vi "TestLoadImages.vi"() -> ()   [LabVIEW 2022 SP3]
uses:
  <vilib>/vision/NI_Vision_Development_Module.lvlib
panel:
  out "ImageMain 7":T1(plugin-control)
  in  "path":path
  out "ImageMain 6":T1(plugin-control)
  out "ImageMain 5":T1(plugin-control)
  out "ImageMain 4":T1(plugin-control)
  out "ImageMain 3":T1(plugin-control)
  out "ImageMain 2":T1(plugin-control)
  # "M:\\DigiLens-1276\\Printer Recipe Files\\Recipe_Patterns\\CalibrationPrints\\Strip Weights\\IP\\SW_IP2.bmp"
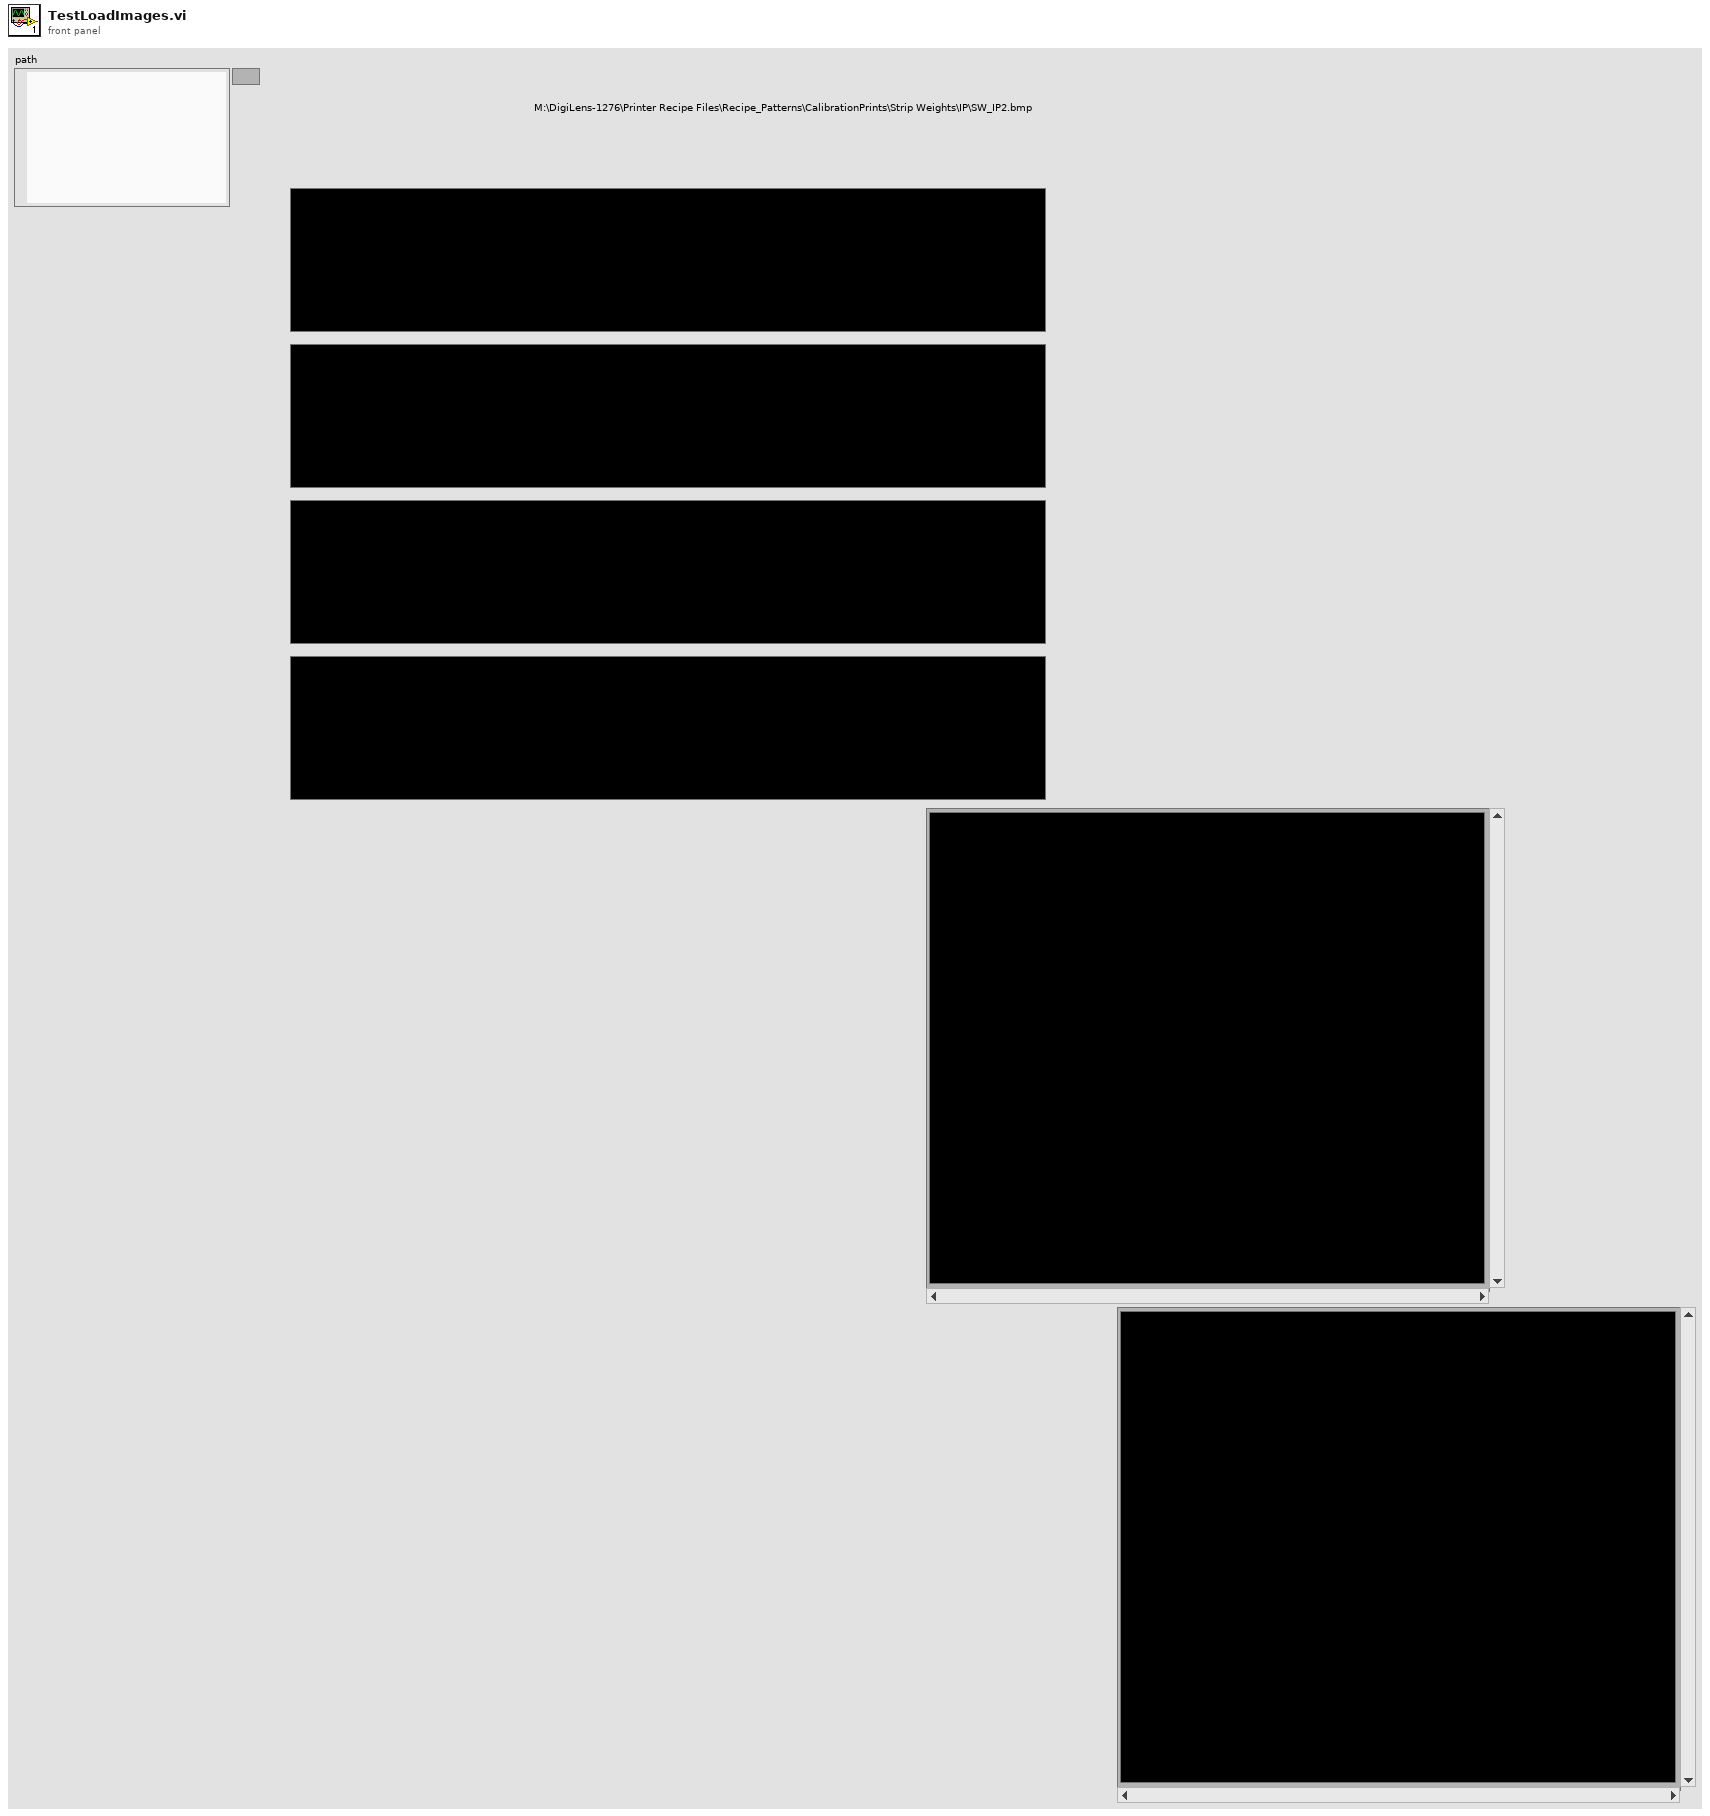
[diagram p1: front panel]
types:
  T1 = typedef "IMAQ Image.ctl" = refnum<image>
  T2 = typedef "Image Type" = u32
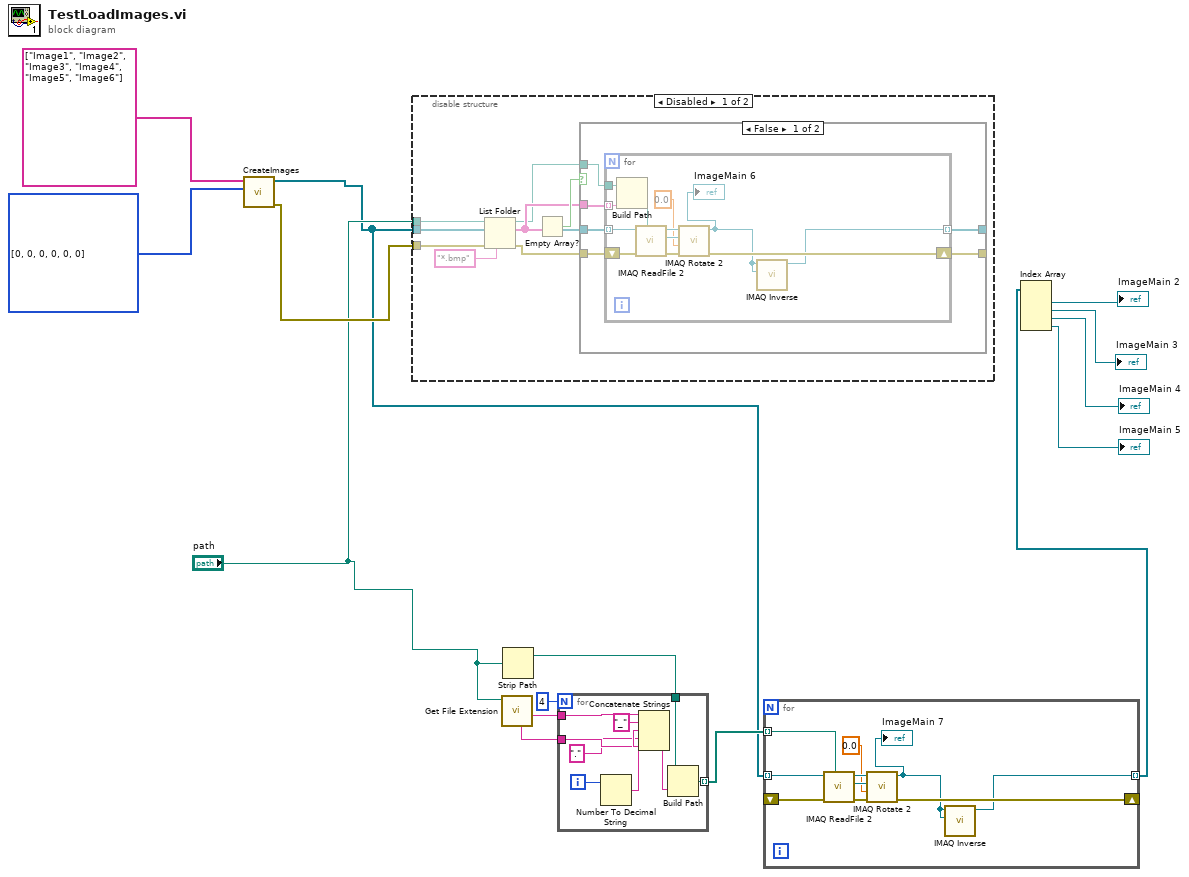
[diagram p0: block diagram]
diagram:
  w15 = T2[] [0, 0, 0, 0, 0, 0] items=["Grayscale (U8)", "Grayscale (I16)", "Grayscale (SGL)", "Complex (CSG)", "RGB (U32)", "HSL (U32)", "RGB (U64)", "Grayscale (U16)"]
  n1 = call "CreateImages.vi"("Array 3"=w15, "Array in"=string[] ["Image1", "Image2", "Image3", "Image4", "Image5", "Image6"]) -> ("error in (no error) 2"=w13:errorcluster, "Array out"=w2:T1[])  [unwired: 8 in]
  n2 = disable-structure shown="Disabled" {
    disable-tunnel: w13 -> [w18 _]
    disable-tunnel: "path" -> [w17 _]
    disable-tunnel: w2 -> [w16 _]
    frame Disabled {
      n3 = List Folder(path=w17, pattern="*.bmp", error in=w18) -> (path out=w19:path, filenames=w21:string[], error out=w20:errorcluster)  [unwired: 1 in, 1 out]
      n4 = Empty Array?(array=w21) -> (empty?=w22:bool)
      n5 = case shown="False" w22 {
        tunnel: w21 -> [w29 _]
        tunnel: w16 -> [w28 w42]
        tunnel: w19 -> [w27 _]
        tunnel: w20 -> [w26 w41]
        tunnel: [w25 w42] -> _
        tunnel: [w24 w41] -> _
        frame False {
          n6 = for {
            tunnel: w29 -> [w40] mode=indexing
            tunnel: w28 -> [w37] mode=indexing
            tunnel: w27 -> [w39]
            shift-right: [w32] -> w24
            shift-left: w26 -> [w36]
            tunnel: [w30] -> w25 mode=indexing
            n7 = Build Path(base path=w39, name or relative path=w40) -> (appended path=w38:path)
            n8 = call "IMAQ ReadFile 2"("File Path"=w38, "error in (no error)"=w36, "Image"=w37) -> ("error out"=w33:errorcluster, "Image Out"=w35:T1)  [unwired: 4 in, 3 out]
            n9 = call "IMAQ Rotate 2"("error in (no error)"=w33, "Angle (degrees)"=0.0, "Image Dst"=w35, "Image Src"=w35) -> ("error out"=w32:errorcluster, "Image Dst Out"=w31:T1)  [unwired: 6 in]
            "ImageMain 6" <- w31
            n10 = call "IMAQ Inverse"("Image Mask"=w31, "Image Src"=w31) -> ("Image Dst Out"=w30:T1)  [unwired: 8 in, 1 out]
          }
        }
        frame True {
        }
      }
    }
    frame Enabled {
    }
  }
  n11 = call <vilib>:"Get File Extension.vi"("file"="path") -> ("filename without extension"=w7:string, "unmodified file extension"=w6:string)  [unwired: 6 in, 3 out]
  n12 = Strip Path(path="path") -> (stripped path=w5:path)  [unwired: 1 out]
  n13 = for {
    N: 4 -> [_]
    tunnel: w7 -> [w51]
    tunnel: w6 -> [w48]
    tunnel: w5 -> [w46]
    tunnel: [w44] -> w3 mode=indexing
    i -> [w50]
    n14 = Number To Decimal String(number=w50) -> (decimal integer string=w49:string)  [unwired: 1 in]
    n15 = Concatenate Strings(w51, "_" ("string"), w49, "." ("string"), w48) -> (w45:string)
    n16 = Build Path(base path=w46, name or relative path=w45) -> (appended path=w44:path)
  }
  n17 = for {
    tunnel: w2 -> [w60] mode=indexing
    tunnel: w3 -> [w52] mode=indexing
    shift-right: [w55] -> _
    shift-left: _ -> [w59]
    tunnel: [w53] -> w1 mode=indexing
    n18 = call "IMAQ ReadFile 2"("File Path"=w52, "error in (no error)"=w59, "Image"=w60) -> ("error out"=w56:errorcluster, "Image Out"=w58:T1)  [unwired: 4 in, 3 out]
    n19 = call "IMAQ Rotate 2"("error in (no error)"=w56, "Angle (degrees)"=0.0, "Image Dst"=w58, "Image Src"=w58) -> ("error out"=w55:errorcluster, "Image Dst Out"=w54:T1)  [unwired: 6 in]
    "ImageMain 7" <- w54
    n20 = call "IMAQ Inverse"("Image Mask"=w54, "Image Src"=w54) -> ("Image Dst Out"=w53:T1)  [unwired: 8 in, 1 out]
  }
  n21 = Index Array(array=w1) -> (element #1=→"ImageMain 2":T1, element #2=→"ImageMain 3":T1, element #3=→"ImageMain 4":T1, element #4=→"ImageMain 5":T1)  [unwired: 4 in]
